vi "PPCS_SIM_SIM_MODULE_EXECUTE.vi"(6 "FPGA_Time_Seconds":dbl=-1.0, 7 "Module Index":i32, 8 "error in (no error)":errorcluster, 9 "Battery Voltage":dbl) -> (0 "error out":errorcluster, 1 "Abs Current":dbl, 2 "Swerve Distance_Radians":dbl, 3 "Wheel Distance_Meters":dbl)   [LabVIEW 2019]
uses:
  <vilib>/Rock Robotics/WPI/ThirdParty/JAS_Junk/TrajLib/Enum/DCMOTOR_TYPES_ENUM.ctl
  PPCS_SIM_SIM_Globals.vi
  <vilib>/Rock Robotics/WPI/ThirdParty/JAS_Junk/TrajLib/Trajectory_Library.lvlib
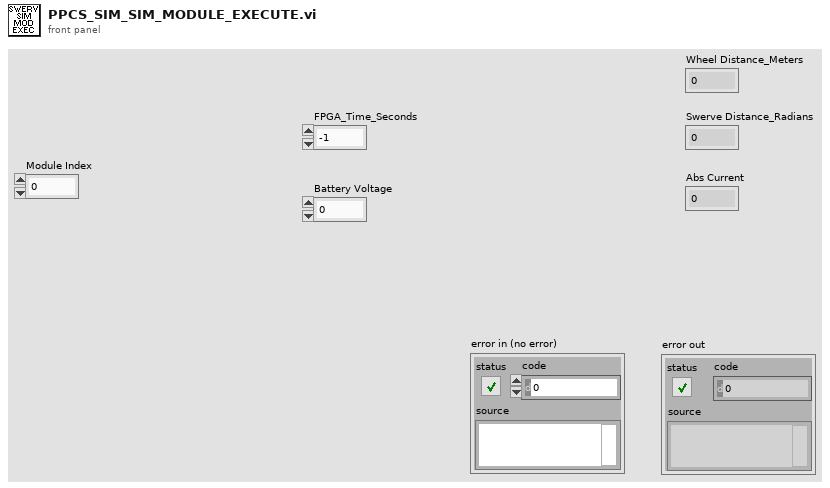
[diagram p1: front panel]
types:
  T1 = typedef "Trajectory_Library.lvlib/DCMOTOR_TYPES_ENUM.ctl" = enum16{"CIM", "AndyMark 9015", "Andy Mark RS 775 125", "Bag", "BaneBots RS 550", "BaneBots RS 775", "Falcon 500", "Mini CIM", "NEO", "NEO 550", "Romi BuiltIn", "Vex 775 Pro", "Snow Blower AM 2235A", "Bosch Seat AM 3493", "Falcon 500 FOC", "Kraken X60", "Kraken X60 FOC", "NEO Vortex"}
  T2 = cluster{"Swerve Motor Device Index":i32, "Drive Motor Device Index":i32, "Swerve Encoder Device Index":i32, "Drive Encoder Device Index":i32, "Drive DistPerzcount":dbl, "SwerveRadPerCount":dbl}[]
  T3 = cluster{"Swerve Motor Device Index":i32, "Drive Motor Device Index":i32, "Swerve Encoder Device Index":i32, "Drive Encoder Device Index":i32, "Drive DistPerzcount":dbl, "SwerveRadPerCount":dbl}
  T4 = typedef "Trajectory_Library.lvlib/LINEAR_SYSTEM_ID_DCMOTOR_MODEL.ctl" = cluster{"DCMOTOR_TYPES":T1, "Num Motors":i32, "Gearing":dbl, "MOI kgm2":dbl}
  T5 = typedef "Trajectory_Library.lvlib/DCMOTOR_SIM_SIMULATION_PARAMS.ctl" = cluster{"Pos Sim Std Dev Rotations":dbl, "Vel Sim Std Dev RPM":dbl}
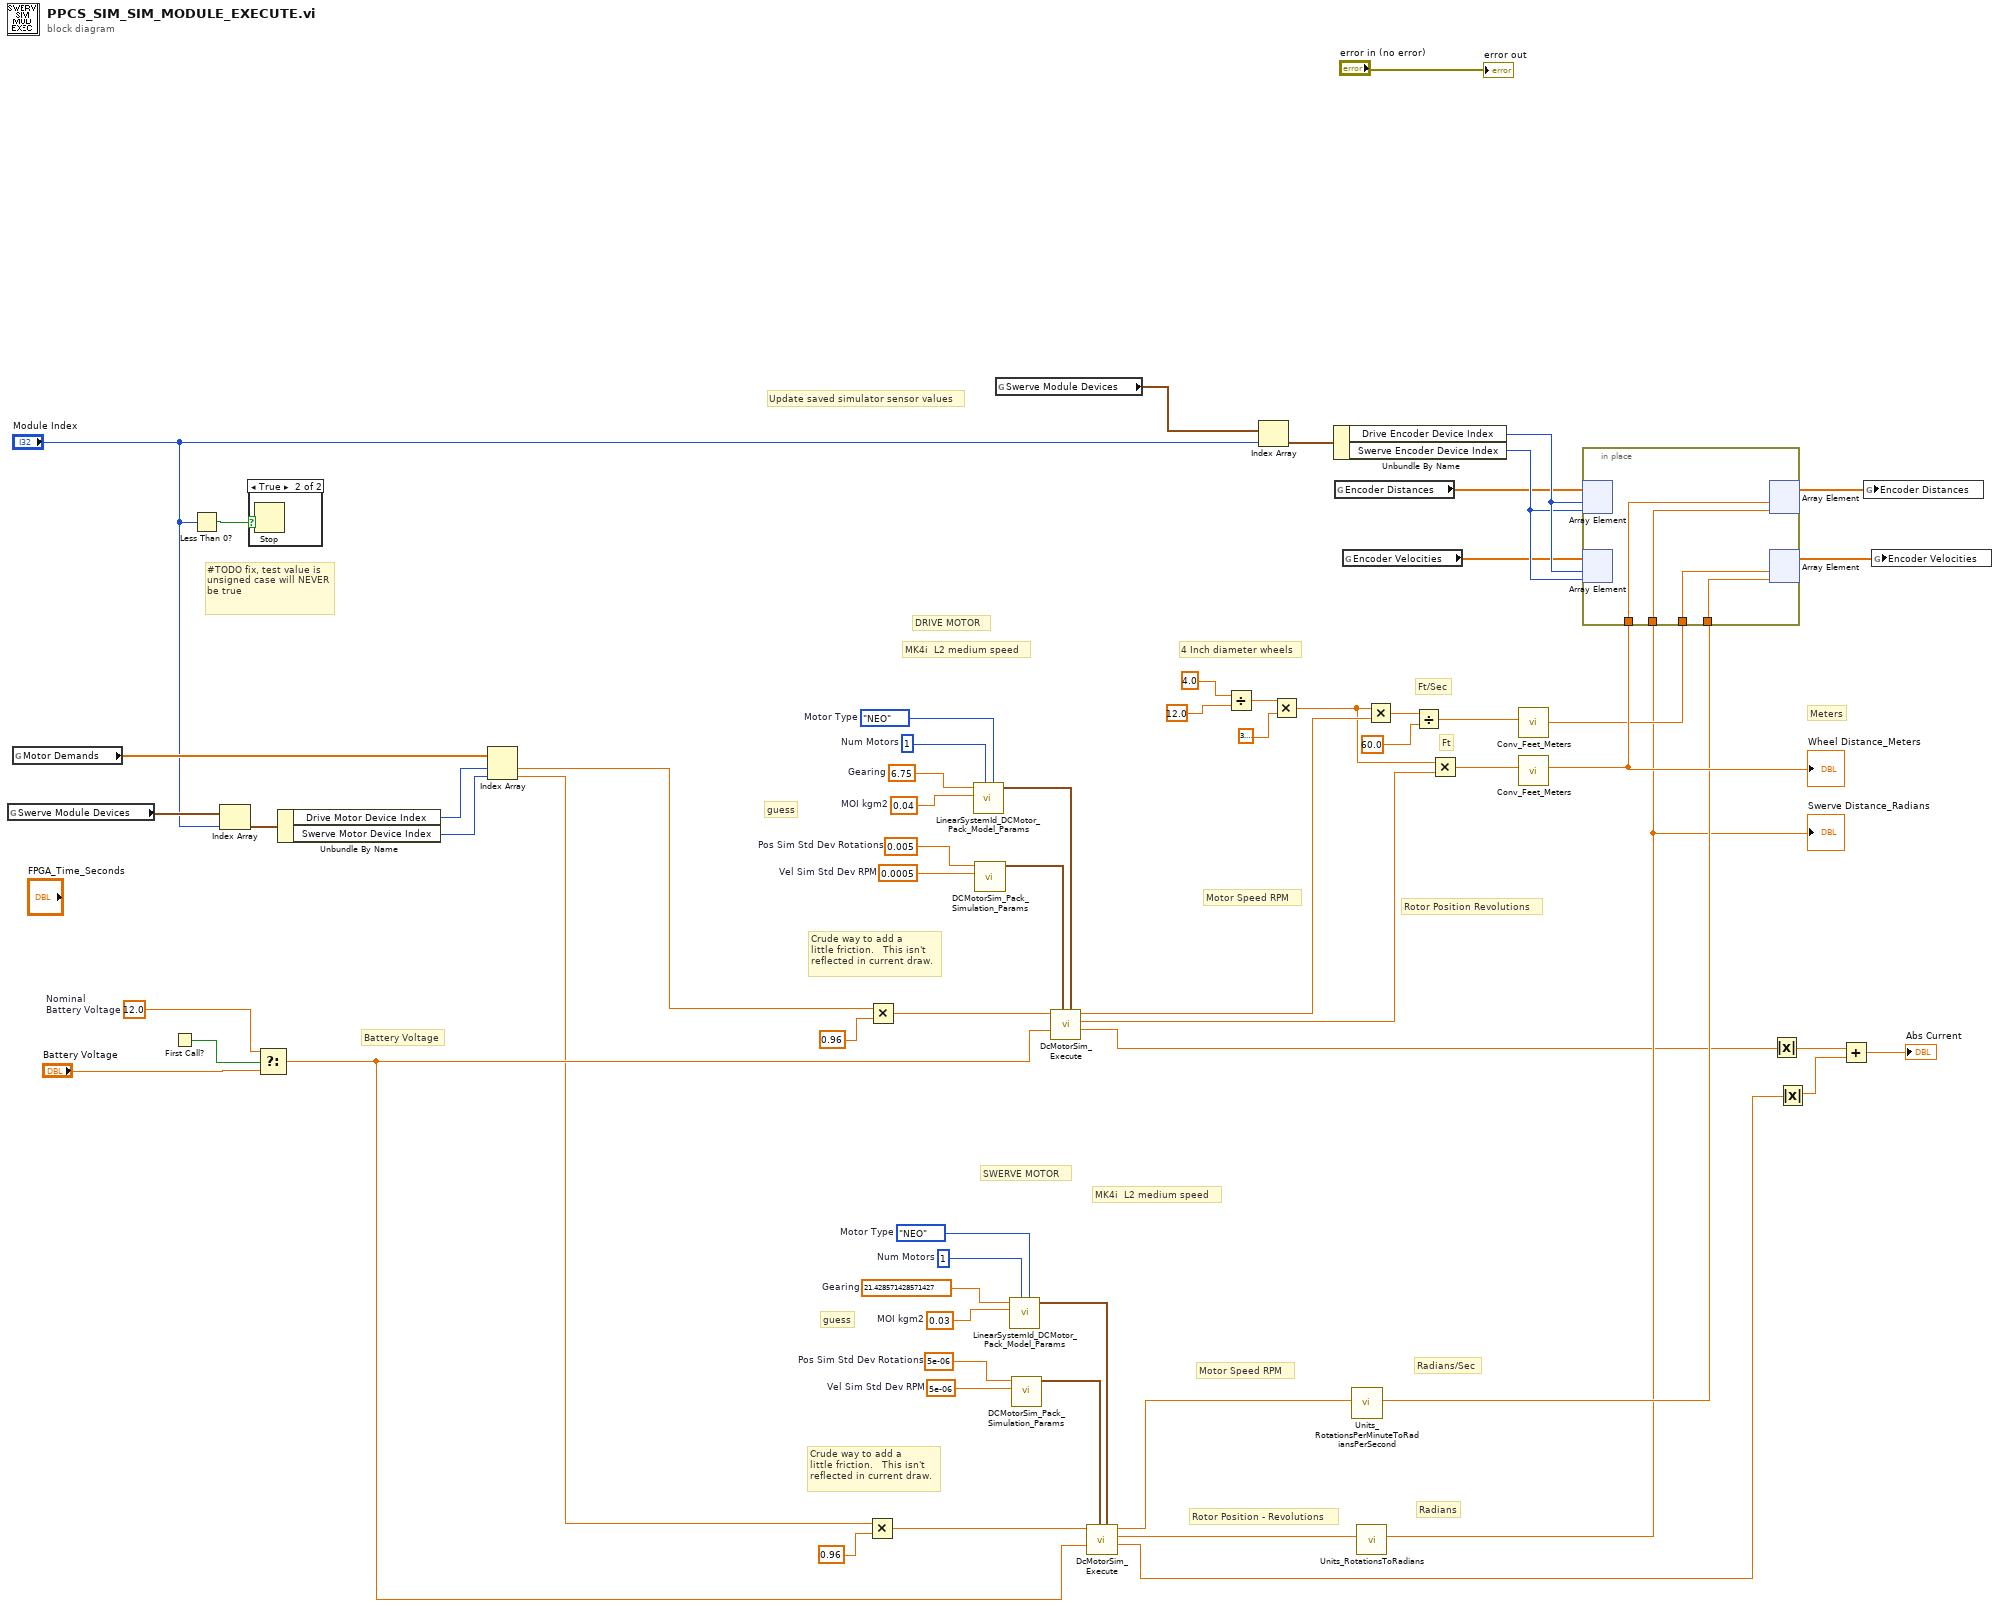
[diagram p0: block diagram]
diagram:
  w32 = 0.005  # Pos Sim Std Dev Rotations
  w33 = 0.0005  # Vel Sim Std Dev RPM
  w36 = 6.75  # Gearing
  w37 = 0.04  # MOI kgm2
  w38 = 1  # Num Motors
  w39 = DCMOTOR_TYPES_ENUM."NEO"  # Motor Type
  w40 = 5e-06  # Pos Sim Std Dev Rotations
  w41 = 5e-06  # Vel Sim Std Dev RPM
  w44 = 21.428571428571427  # Gearing
  w45 = 0.03  # MOI kgm2
  w46 = 1  # Num Motors
  w47 = DCMOTOR_TYPES_ENUM."NEO"  # Motor Type
  w30 = 12.0  # Nominal Battery Voltage
  # "Crude way to add a \nlittle friction.   This isn't\nreflected in current draw."
  # "Crude way to add a \nlittle friction.   This isn't\nreflected in current draw."
  # "Battery Voltage"
  # "4 Inch diameter wheels"
  # "Radians"
  # "Radians/Sec"
  # "guess"
  # "guess"
  # "Ft/Sec"
  # "Ft"
  # "MK4i  L2 medium speed"
  # "MK4i  L2 medium speed"
  # "Rotor Position Revolutions"
  # "Motor Speed RPM"
  # "Rotor Position - Revolutions"
  # "Motor Speed RPM"
  # "SWERVE MOTOR"
  # "DRIVE MOTOR"
  # "Update saved simulator sensor values"
  # "#TODO fix, test value is unsigned case will NEVER be true"
  # "Meters"
  n1 = global read "PPCS_SIM_SIM_Globals.vi" "Swerve Module Devices"() -> (w54:T2)
  n2 = global read "PPCS_SIM_SIM_Globals.vi" "Motor Demands"() -> (w52:dbl[])
  n3 = First Call?() -> (First Call?: T/F=w31:bool)
  n4 = Less Than 0?(x="Module Index") -> (x < 0?=w63:bool)
  n5 = Index Array(array=w54, index="Module Index") -> (element=w53:T3)
  n6 = case shown="True" w63 {
    frame False {
    }
    frame True {
      n7 = Stop() -> ()  [unwired: 1 in]
    }
  }
  n8 = Select(t=w30, s=w31, f="Battery Voltage") -> (s? t:f=w9:dbl)
  n9 = Unbundle By Name(w53) -> ("Drive Motor Device Index"=w51:i32, "Swerve Motor Device Index"=w50:i32)
  n10 = Index Array(array=w52, index #1=w51, index #2=w50) -> (element #1=w2:dbl, element #2=w6:dbl)
  n11 = Multiply(x=w6, y=0.96) -> (x*y=w4:dbl)
  n12 = Multiply(x=w2, y=0.96) -> (x*y=w1:dbl)
  n13 = call <vilib>:"LinearSystemId_DCMotor_Pack_Model_Params.vi"("DCMOTOR_TYPES"=w39, "Num Motors"=w38, "MOI kgm2"=w37, "Gearing"=w36) -> ("LinearSystem_ID_DCMotor_Model"=w35:T4)  [unwired: 7 in]
  n14 = call <vilib>:"DCMotorSim_Pack_Simulation_Params.vi"("Vel Sim Std Dev RPM"=w33, "Pos Sim Std Dev Rotations"=w32) -> ("DCMOTOR_Sim_Simulation_Params"=w34:T5)  [unwired: 9 in]
  n15 = global read "PPCS_SIM_SIM_Globals.vi" "Swerve Module Devices"() -> (w62:T2)
  n16 = call <vilib>:"LinearSystemId_DCMotor_Pack_Model_Params.vi"("DCMOTOR_TYPES"=w47, "Num Motors"=w46, "MOI kgm2"=w45, "Gearing"=w44) -> ("LinearSystem_ID_DCMotor_Model"=w43:T4)  [unwired: 7 in]
  n17 = call <vilib>:"DCMotorSim_Pack_Simulation_Params.vi"("Vel Sim Std Dev RPM"=w41, "Pos Sim Std Dev Rotations"=w40) -> ("DCMOTOR_Sim_Simulation_Params"=w42:T5)  [unwired: 9 in]
  n18 = call <vilib>:"DcMotorSim_Execute.vi"("DCMotor_Model _Params"=w35, "DCMOTORSim_Simulation_Params"=w34, "Battery Voltage"=w9, "Motor Dmd (CO)"=w1) -> ("Motor Current"=w11:dbl, "Position_Rotations"=w23:dbl, "Velocity_RPM"=w25:dbl)  [unwired: 3 in, 2 out]
  n19 = call <vilib>:"DcMotorSim_Execute.vi"("DCMotor_Model _Params"=w43, "DCMOTORSim_Simulation_Params"=w42, "Battery Voltage"=w9, "Motor Dmd (CO)"=w4) -> ("Motor Current"=w12:dbl, "Position_Rotations"=w14:dbl, "Velocity_RPM"=w16:dbl)  [unwired: 3 in, 2 out]
  n20 = Divide(x=4.0, y=12.0) -> (x/y=w27:dbl)
  n21 = Index Array(array=w62, index="Module Index") -> (element=w61:T3)
  n22 = Multiply(x=w27, y=3.141592653589793) -> (x*y=w24:dbl)
  n23 = Unbundle By Name(w61) -> ("Drive Encoder Device Index"=w60:i32, "Swerve Encoder Device Index"=w59:i32)
  n24 = global read "PPCS_SIM_SIM_Globals.vi" "Encoder Distances"() -> (w58:dbl[])
  n25 = global read "PPCS_SIM_SIM_Globals.vi" "Encoder Velocities"() -> (w57:dbl[])
  n26 = call <vilib>:"Units_RotationsPerMinuteToRadiansPerSecond.vi"("RotationsPerMinute"=w16) -> ("RadiansPerSecond"=w15:dbl)  [unwired: 10 in]
  n27 = call <vilib>:"Units_RotationsToRadians.vi"("Rotations"=w14) -> ("Radians"=w13:dbl)  [unwired: 10 in]
  "Swerve Distance_Radians" <- w13
  n28 = Multiply(x=w24, y=w25) -> (x*y=w22:dbl)
  n29 = Divide(x=w22, y=60.0) -> (x/y=w20:dbl)
  n30 = Multiply(x=w24, y=w23) -> (x*y=w19:dbl)
  n31 = call <vilib>:"Conv_Feet_Meters.vi"("Feet"=w20) -> ("Meters"=w17:dbl)  [unwired: 10 in]
  n32 = call <vilib>:"Conv_Feet_Meters.vi"("Feet"=w19) -> ("Meters"=w18:dbl)  [unwired: 10 in]
  "Wheel Distance_Meters" <- w18
  n33 = in-place {
    in-place-border: w13 -> [w65]
    in-place-border: w18 -> [w66]
    in-place-border: w17 -> [w68]
    in-place-border: w15 -> [w67]
    n34 = in-place-array #1(w58, w60, w59) -> ()  [unwired: 2 out]
    n35 = in-place-array #2(w57, w60, w59) -> ()  [unwired: 2 out]
    n36 = in-place-array #1(w66, w65) -> (w56:dbl[])  [unwired: 2 out]
    n37 = in-place-array #2(w68, w67) -> (w55:dbl[])  [unwired: 2 out]
  }
  n38 = Absolute Value(x=w11) -> (abs(x)=w8:dbl)
  n39 = Absolute Value(x=w12) -> (abs(x)=w7:dbl)
  n40 = Add(x=w8, y=w7) -> (x+y=→"Abs Current":dbl)
  n41 = global write "PPCS_SIM_SIM_Globals.vi" "Encoder Distances"(w56) -> ()
  n42 = global write "PPCS_SIM_SIM_Globals.vi" "Encoder Velocities"(w55) -> ()
  "error out" <- "error in (no error)"
